vi "_read_CLNA_params.vi"(10 "Control":T1={"GPIB_ATT"="28", "6501Dev#"=1, "GPIB_SP"="18", "GPIB_PM"="13", "GPIB_DSA"="11", "GPIB_DMM (TPD)"="23", "GPIB_MPI"="2", "mortor設定"=[{"Axis"=0, "ID"=0, "HIspeed"=200.0, "LOspeed"=100.0, "ACCEL(ms)"=100.0, "Sratio"=50.0, "フリーラン\n"=FALSE, "文字列"="DSB HOT/COLD"}, {"Axis"=1, "ID"=0, "HIspeed"=4.0, "LOspeed"=4.0, "ACCEL(ms)"=100.0, "Sratio"=50.0, "フリーラン\n"=TRUE, "文字列"="SubMM Att"}, {"Axis"=0, "ID"=0, "HIspeed"=200.0, "LOspeed"=100.0, "ACCEL(ms)"=100.0, "Sratio"=50.0, "フリーラン\n"=TRUE, "文字列"="MPI Port1"}, {"Axis"=1, "ID"=0, "HIspeed"=200.0, "LOspeed"=100.0, "ACCEL(ms)"=100.0, "Sratio"=50.0, "フリーラン\n"=TRUE, "文字列"="MPI Port2"}, {"Axis"=1, "ID"=0, "HIspeed"=200.0, "LOspeed"=100.0, "ACCEL(ms)"=100.0, "Sratio"=50.0, "フリーラン\n"=TRUE, "文字列"="gainComp"}], "DATAパス"=path "C:/Documents and Settings/?澤佳?/デスクトップ/data/プロトカ?トリッジ/110113_protoC4-9/110127_mixtest", "DBパス "=path "Z:/band10/Labview_ALMA/MIX95/test", "comment"="mix10test", "ColdCarts"="003601", "Th"=300.0, "Tc"=77.0, "Set_SIS_volt"=2.0999999046325684, "Offset"=0.0, "control"=0, "FreqLO"=874.0, "Set_Mag_Cur"=800.0, "MPI offset(mm)"=22.962, "HOT/COLD"=0} {"HOT/COLD" items=["DSB", "SBR (Cart.)", "GainComp", "SBR (MIX)"]; "control" items=["CLOSE LOOP", "OPEN LOOP", "Not Control"]}, 11 "Bias_LO_equip":T3={"Node address"=19, "CAN Interface"="CAN1", "Cartridge band"=10, "Slave Node in"={"Address"=19, "Serial Number"=[16, 71, 55, 76, 1, 8, 0, -15]}, "ObjHandle out"=214106176, "POL"=1, "sb"=1, "GPIB_SM (SIS S,V)"="24", "GPIB_DMM (SIS I)"="22", "GPIB_SM (MAG I) "="25", "GPIB_SG(LO)"="19", "GPIB_PW (PAMP) "="6", "GPIB_TMP1(8ch)"="12", "GPIB_TMP2(2ch)  "="13", "WCA_avg"=10, "Rsen"=10.0, "BiasModule"=1, "LOModule "=5, "WCA_LO_FREQ_SET"={"YTO Low freq. [GHz]"=14.42, "YTO High freq. [GHz]"=17.7, "Kvco"=1, "Lock Pol."=0, "SET LO FREQ"=96.22222, "Multiplier"=6.0, "YTO (HEX)"=2014, "YTO ( FREQ)"=16.033167, "NULL PLL INTEGRATOR"=FALSE}, "Res for"=0} {"Res for" items=["none", "series res", "parallel res"]; "WCA_LO_FREQ_SET"."YTO ( FREQ)" min=25 max=150 step=0.0001 format="%.3f"; "WCA_LO_FREQ_SET"."Multiplier" min=3 max=6 step=3; "WCA_LO_FREQ_SET"."SET LO FREQ" min=25 max=150 step=0.0001 format="%.3f"; "WCA_LO_FREQ_SET"."Lock Pol." items=["Lower", "Upper"]; "WCA_LO_FREQ_SET"."Kvco" items=["7.5MHz/V", "15MHz/V"]; "WCA_LO_FREQ_SET"."YTO High freq. [GHz]" format="%.3f"; "WCA_LO_FREQ_SET"."YTO Low freq. [GHz]" format="%.3f"; "LOModule" items=["Manual Gunn+PAMP"=0, "PLL GUNN+PAMP"=5, "B10Lab LO"=1, "WCA LO"=2, ""=3, "YIG発信器"=4, "none"=99]; "BiasModule" items=["B10Lab Bias"=0, "WCA BiasModule"=1, "none"=99]; "Slave Node in"."Serial Number" format="%.0x"; "Slave Node in"."Address" format="%.0x"; "Cartridge band" max=10 step=1; "Node address" format="%.0x"}) -> (3 "文字列":string="PreampParam, 3.65, 874.00, 2011-02-04  19:50:11, 1.40, 0.00, 0.00,  12.05, 0.00, 0.02,  -1.53, 4.91, 4.91,")   [LabVIEW 2017]
uses:
  WCA_NAOJ_sub_vi/WCA_Global.vi
panel:
  in  "CLNA_SET":T2={"CLNA State"=1, "SET POL0 LNA1 STAGE1 DRAIN V"=0.0, "SET POL0 LNA1 STAGE1 DRAIN C"=0.0, "SET POL0 LNA1 STAGE2 DRAIN V"=0.0, "SET POL0 LNA1 STAGE2 DRAIN C"=0.0, "SET POL0 LNA1 STAGE3 DRAIN V"=0.0, "SET POL0 LNA1 STAGE3 DRAIN C"=0.0} {"SET POL0 LNA1 STAGE3 DRAIN C" min=0 max=20 step=0.01 format="%.2f"; "SET POL0 LNA1 STAGE3 DRAIN V" min=0 max=3 step=0.01 format="%.2f"; "SET POL0 LNA1 STAGE2 DRAIN C" min=0 max=20 step=0.01 format="%.2f"; "SET POL0 LNA1 STAGE2 DRAIN V" min=0 max=3 step=0.01 format="%.2f"; "SET POL0 LNA1 STAGE1 DRAIN C" min=0 max=20 step=0.01 format="%.2f"; "SET POL0 LNA1 STAGE1 DRAIN V" min=0 max=3 step=0.01 format="%.2f"; "CLNA State" items=["Disabled", "Enabled"]}
  out "Link済み":bool
  # "Vd [V]"
  # "Id [mA]"
  # "Stage 1"
  # "Stage 2"
  # "Stage 3"
  # "LO freq. [GHz]"
  # "YTO LOW\n/High Freq."
  # "ZERO Intgrtr"
  # "Node Address"
  # "Serial Number"
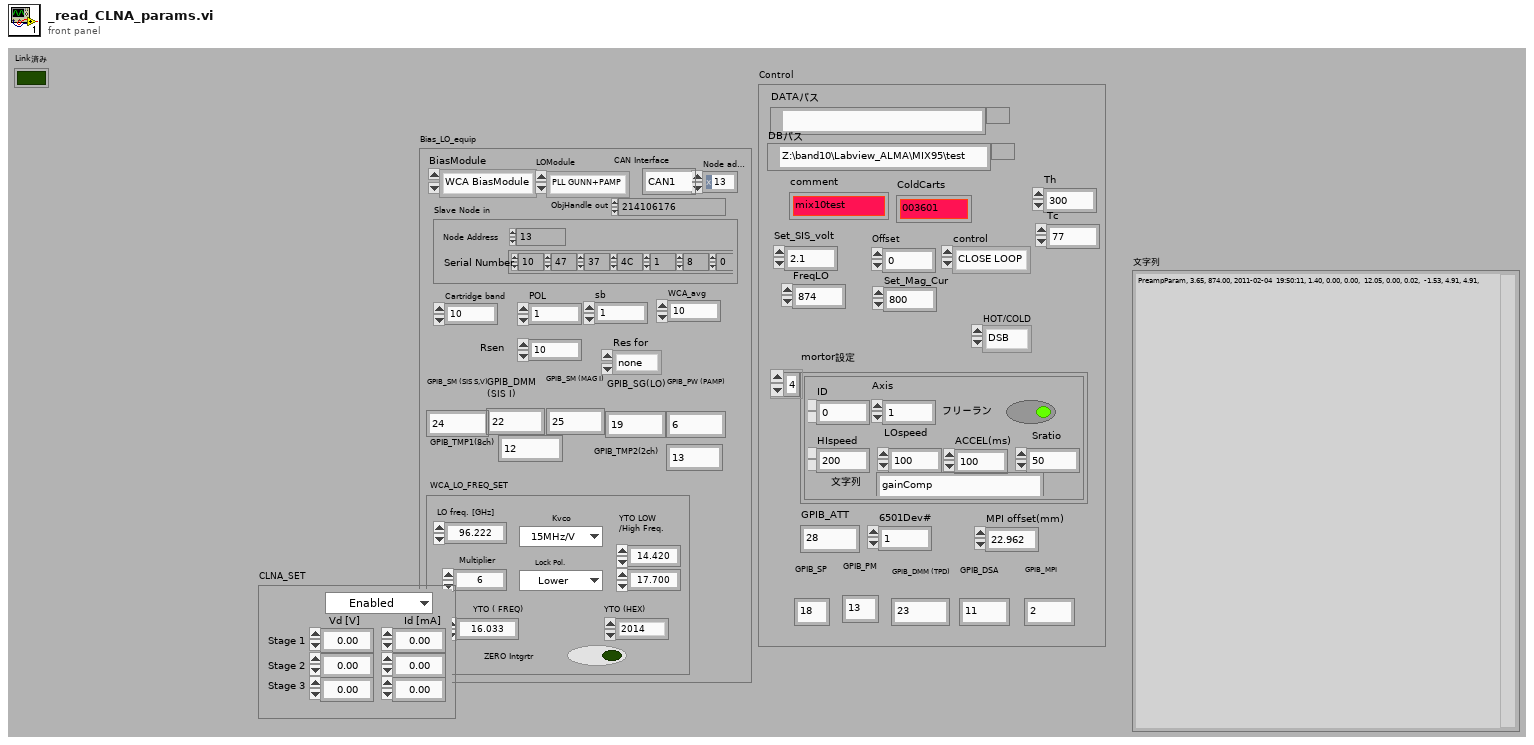
[diagram p1: front panel]
types:
  T1 = cluster{"GPIB_ATT":string, "6501Dev#":i16, "GPIB_SP":string, "GPIB_PM":string, "GPIB_DSA":string, "GPIB_DMM (TPD)":string, "GPIB_MPI":string, "mortor設定":cluster{"Axis":i16, "ID":i16, "HIspeed":dbl, "LOspeed":dbl, "ACCEL(ms)":dbl, "Sratio":dbl, "フリーラン\n":bool, "文字列":string}[], "DATAパス":path, "DBパス ":path, "comment":string, "ColdCarts":string, "Th":dbl, "Tc":dbl, "Set_SIS_volt":dbl, "Offset":dbl, "control":u16, "FreqLO":dbl, "Set_Mag_Cur":dbl, "MPI offset(mm)":dbl, "HOT/COLD":u16}
  T2 = cluster{"CLNA State":u8, "SET POL0 LNA1 STAGE1 DRAIN V":sgl, "SET POL0 LNA1 STAGE1 DRAIN C":sgl, "SET POL0 LNA1 STAGE2 DRAIN V":sgl, "SET POL0 LNA1 STAGE2 DRAIN C":sgl, "SET POL0 LNA1 STAGE3 DRAIN V":sgl, "SET POL0 LNA1 STAGE3 DRAIN C":sgl}
  T3 = cluster{"Node address":u16, "CAN Interface":string, "Cartridge band":u32, "Slave Node in":cluster{"Address":i16, "Serial Number":i8[]}, "ObjHandle out":u32, "POL":u32, "sb":u32, "GPIB_SM (SIS S,V)":string, "GPIB_DMM (SIS I)":string, "GPIB_SM (MAG I) ":string, "GPIB_SG(LO)":string, "GPIB_PW (PAMP) ":string, "GPIB_TMP1(8ch)":string, "GPIB_TMP2(2ch)  ":string, "WCA_avg":i32, "Rsen":dbl, "BiasModule":u16, "LOModule ":u16, "WCA_LO_FREQ_SET":cluster{"YTO Low freq. [GHz]":sgl, "YTO High freq. [GHz]":sgl, "Kvco":u16, "Lock Pol.":u16, "SET LO FREQ":sgl, "Multiplier":sgl, "YTO (HEX)":u16, "YTO ( FREQ)":sgl, "NULL PLL INTEGRATOR":bool}, "Res for":u16}
  T4 = cluster{"Pol0 LNA1 S1 Drain V [V]":sgl, "Pol0 LNA1 S1 Drain C [mA]":sgl, "Pol0 LNA1 S1 Gate V [V]":sgl, "Pol0 LNA1 S2 Drain V [V]":sgl, "Pol0 LNA1 S2 Drain C [mA]":sgl, "Pol0 LNA1 S2 Gate V [V]":sgl, "Pol0 LNA1 S3 Drain V [V]":sgl, "Pol0 LNA1 S3 Drain C [mA]":sgl, "Pol0 LNA1 S3 Gate V [V]":sgl, "Pol0 LNA1 State":enum16{"Disabled", "Enabled"}}
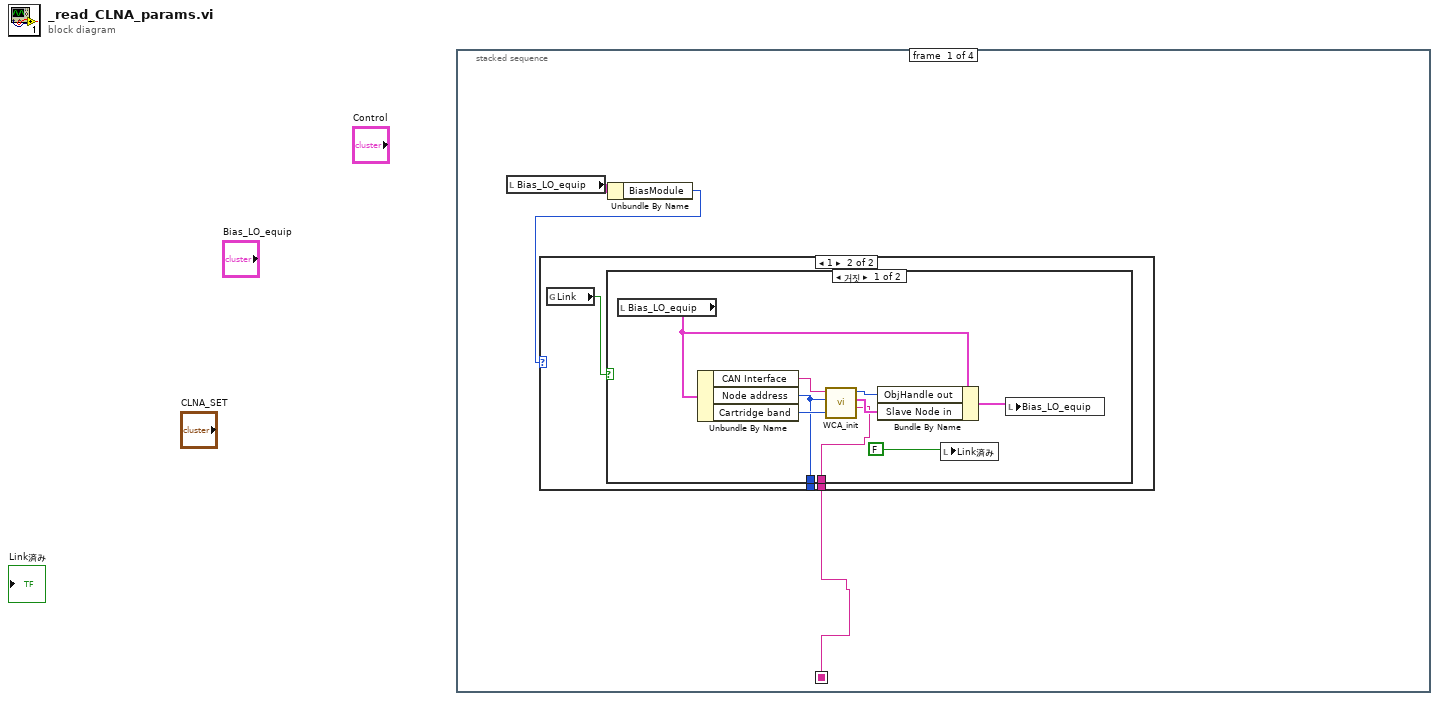
[diagram p0: block diagram]
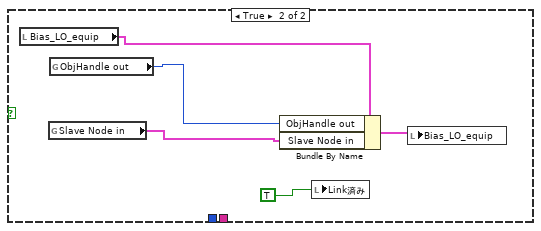
[diagram p3: hidden frame]
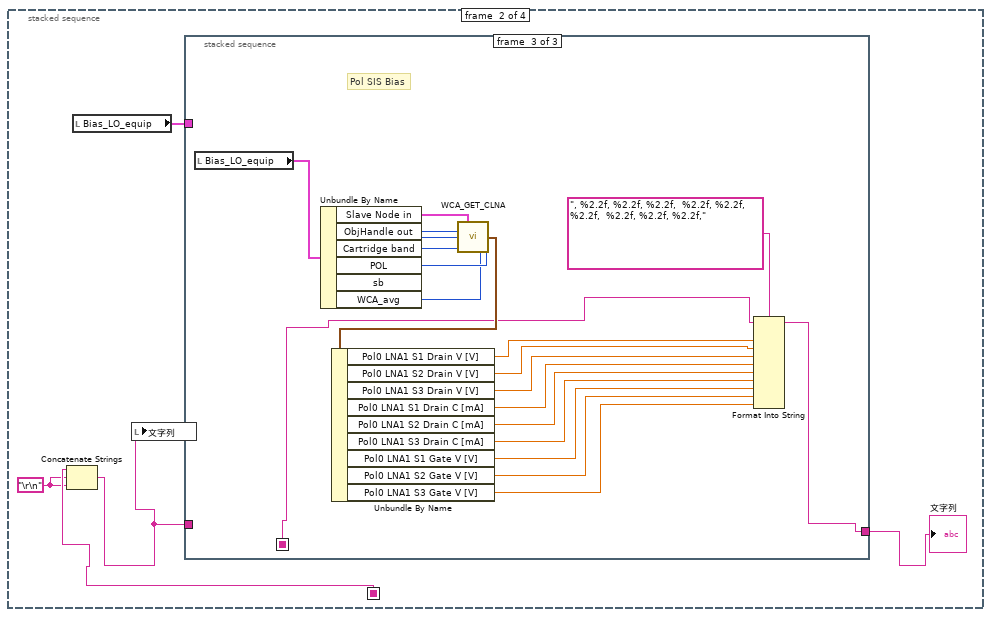
[diagram p4: hidden frame]
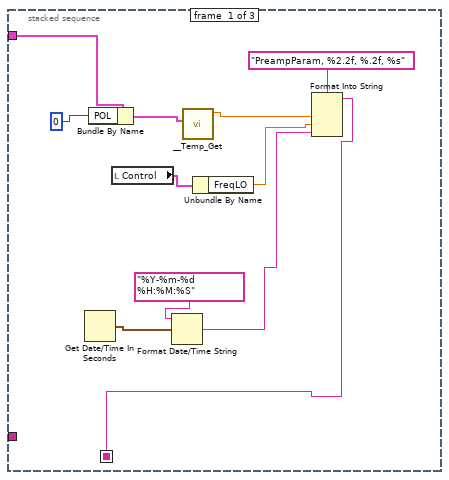
[diagram p5: hidden frame]
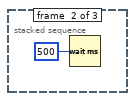
[diagram p6: hidden frame]
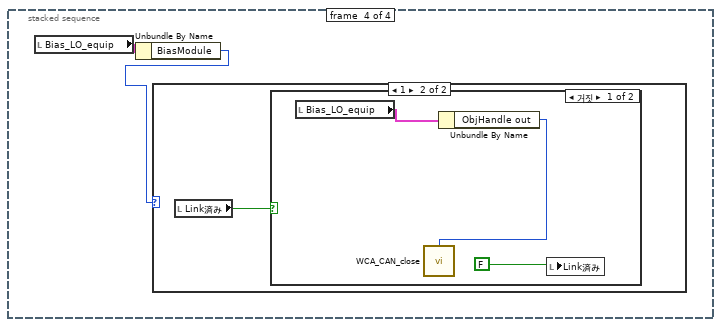
[diagram p8: hidden frame]
diagram:
  n1 = stacked-sequence {
    seq-local: [w1 _ _ _] -> [_ w24 _ _]
    frame #0 {
      n2 = local read "Bias_LO_equip"() -> (w3:T3)
      n3 = Unbundle By Name(w3) -> ("BiasModule"=w2:u16)
      n4 = case shown="1" w2 {
        tunnel: [_ w5] -> w1
        tunnel: [_ w4] -> _
        frame 0, Default {
        }
        frame 1 {
          n5 = global read "WCA_Global.vi" "Link"() -> (w6:bool)
          n6 = case shown="거짓" w6 {
            tunnel: [w7 _] -> w5
            tunnel: [w8 _] -> w4
            frame False {
              n7 = local read "Bias_LO_equip"() -> (w9:T3)
              n8 = Unbundle By Name(w9) -> ("CAN Interface"=w12:string, "Node address"=w8:u16, "Cartridge band"=w11:u32)
              n9 = call "WCA_init.vi"("Cartridge band"=w11, "Node address"=w8, "CAN Interface"=w12) -> ("Detected CAN Nodes."=w7:string, "Slave Node in"=w14:cluster{"Address":i16, "Serial Number":i8[]}, "ObjHandle out"=w15:u32)  [unwired: 4 in, 2 out]
              n10 = Bundle By Name(cluster=w9, "ObjHandle out"=w15, "Slave Node in"=w14) -> (w10:T3)
              n11 = local write "Link済み"(FALSE) -> ()
              n12 = local write "Bias_LO_equip"(w10) -> ()
            }
            frame True {
              n13 = local read "Bias_LO_equip"() -> (w19:T3)
              n14 = global read "WCA_Global.vi" "Slave Node in"() -> (w17:cluster{"Address":i16, "Serial Number":i8[]})
              n15 = global read "WCA_Global.vi" "ObjHandle out"() -> (w18:u32)
              n16 = Bundle By Name(cluster=w19, "ObjHandle out"=w18, "Slave Node in"=w17) -> (w20:T3)
              n17 = local write "Link済み"(TRUE) -> ()
              n18 = local write "Bias_LO_equip"(w20) -> ()
            }
          }
        }
      }
    }
    frame #1 {
      w23 = "\r\n"
      n19 = Concatenate Strings(w24, w23, w23) -> (w22:string)
      n20 = local read "Bias_LO_equip"() -> (w21:T3)
      n21 = local write "文字列"(w22) -> ()
      n22 = stacked-sequence {
        seq-local: [w30 _ _] -> [_ _ w47]
        tunnel: w22 -> [_ _ _]
        tunnel: [_ _ w57] -> w25
        tunnel: w21 -> [w29 _ _]
        frame #0 {
          n23 = Get Date/Time In Seconds() -> (seconds since 1Jan1904=w35:timestamp)
          n24 = Bundle By Name(cluster=w29, "POL"=0) -> (w28:T3)
          n25 = local read "Control"() -> (w33:T1)
          n26 = Format Date/Time String(time format string (%c)="%Y-%m-%d  %H:%M:%S", seconds (now)=w35) -> (date/time string=w31:string)  [unwired: 1 in]
          n27 = call "__Temp_Get.vi"("Bias_LO_equip"=w28) -> ("4K_Temp"=w26:dbl)  [unwired: 8 in, 2 out]
          n28 = Unbundle By Name(w33) -> ("FreqLO"=w32:dbl)
          n29 = Format Into String(format string="PreampParam, %2.2f, %.2f, %s", w26, w32, w31) -> (resulting string=w30:string)  [unwired: 2 in, 1 out]
        }
        frame #1 {
          n30 = Wait (ms)(milliseconds to wait=500) -> ()  [unwired: 1 out]
        }
        frame #2 {
          # "Pol SIS Bias"
          n31 = local read "Bias_LO_equip"() -> (w55:T3)
          n32 = Unbundle By Name(w55) -> ("Slave Node in"=w48:cluster{"Address":i16, "Serial Number":i8[]}, "ObjHandle out"=w53:u32, "Cartridge band"=w52:u32, "POL"=w51:u32, "sb"=w50:u32, "WCA_avg"=w49:i32)
          n33 = call "WCA_GET_CLNA.vi"("Cartridge Band"=w52, "Slave Node in"=w48, "ObjHandle in"=w53, "POL"=w51, "sb"=w50, "avg"=w49) -> ("CLNA_monitor"=w54:T4)  [unwired: 7 in, 2 out]
          n34 = Unbundle By Name(w54) -> ("Pol0 LNA1 S1 Drain V [V]"=w46:sgl, "Pol0 LNA1 S2 Drain V [V]"=w45:sgl, "Pol0 LNA1 S3 Drain V [V]"=w44:sgl, "Pol0 LNA1 S1 Drain C [mA]"=w43:sgl, "Pol0 LNA1 S2 Drain C [mA]"=w42:sgl, "Pol0 LNA1 S3 Drain C [mA]"=w41:sgl, "Pol0 LNA1 S1 Gate V [V]"=w40:sgl, "Pol0 LNA1 S2 Gate V [V]"=w39:sgl, "Pol0 LNA1 S3 Gate V [V]"=w38:sgl)
          n35 = Format Into String(format string=", %2.2f, %2.2f, %2.2f,  %2.2f, %2.2f, %2.2f,  %2.2f, %2.2f, %2.2f,", initial string=w47, w46, w45, w44, w43, w42, w41, w40, w39, w38) -> (resulting string=w57:string)  [unwired: 1 in, 1 out]
        }
      }
      "文字列" <- w25
    }
    frame #2 {
    }
    frame #3 {
      n36 = local read "Bias_LO_equip"() -> (w59:T3)
      n37 = Unbundle By Name(w59) -> ("BiasModule"=w58:u16)
      n38 = case shown="1" w58 {
        frame 0, Default {
        }
        frame 1 {
          n39 = local read "Link済み"() -> (w60:bool)
          n40 = case shown="거짓" w60 {
            frame False {
              n41 = local read "Bias_LO_equip"() -> (w62:T3)
              n42 = Unbundle By Name(w62) -> ("ObjHandle out"=w61:u32)
              n43 = call "WCA_CAN_close.vi"("ObjHandle in"=w61) -> ()  [unwired: 14 in, 1 out]
              n44 = local write "Link済み"(FALSE) -> ()
            }
            frame True {
            }
          }
        }
      }
    }
  }
